vi "Write Data.vi"(0 "comm interface in":refnum<class "RoboRIO I2C.lvclass">, 5 "data":u8[](array[numeric]), 11 "error in":errorcluster) -> (4 "comm interface out":refnum<class "RoboRIO I2C.lvclass">, 15 "error out":errorcluster)   [LabVIEW 2018, in "RoboRIO I2C.lvclass"]
uses:
  RoboRIO I2C.lvclass
  RoboRIO I2C.lvclass/RoboRIO I2C.ctl
panel:
  # "write address is encoded in index 0"
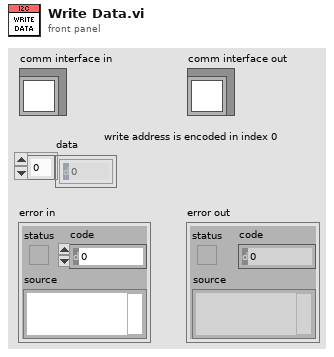
[diagram p1: front panel]
types:
  T1 = typedef "WPI_I2CDevRef.ctl" = cluster{"DevStatus":errorcluster, "Device Address":u8, "Handle":i32, "I2C Bus":T2}
  T2 = typedef "i2c_bus.ctl" = enum16{"I2C On-Board", "I2C MXP", "Invalid"}
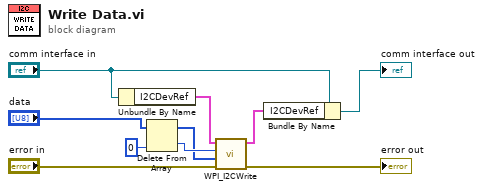
[diagram p0: block diagram]
diagram:
  n1 = Unbundle By Name("comm interface in") -> ("I2CDevRef"=w4:T1)
  n2 = Delete From Array(array="data", index=0) -> (deleted portion=w6:u8, array with subset deleted=w5:u8[])  [unwired: 1 in]
  n3 = call <vilib>:"WPI_I2CWrite.vi"("error in (no error)"="error in", "I2CDataToSend"=w5, "I2CRegister"=w6, "I2CDevRef"=w4) -> ("error out"=→"error out":errorcluster, "I2CDevRef"=w3:T1)  [unwired: 6 in]
  n4 = Bundle By Name(cluster="comm interface in", "I2CDevRef"=w3) -> (→"comm interface out":refnum<class "RoboRIO I2C.lvclass">)
